vi "ExecuteCommand.vi"(8 "error in (no error)":errorcluster, 10 "Command":string, 11 "VISA resource name":refnum<visa-resource-name>) -> (0 "error out":errorcluster, 2 "Response":string, 3 "VISA resource name out":refnum<visa-resource-name>)   [LabVIEW 2018, in "CAEN PSM.lvlib"]
uses:
  CAEN PSM.lvlib
  <vilib>/Instr/_visa.llb/Select Event Type.ctl
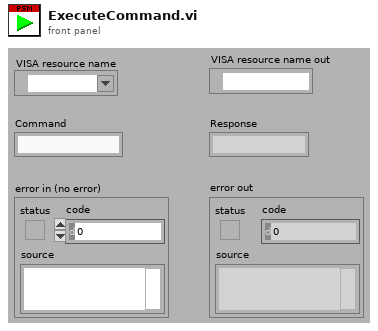
[diagram p1: front panel]
types:
  T1 = typedef "Select Event Type.ctl" = u32
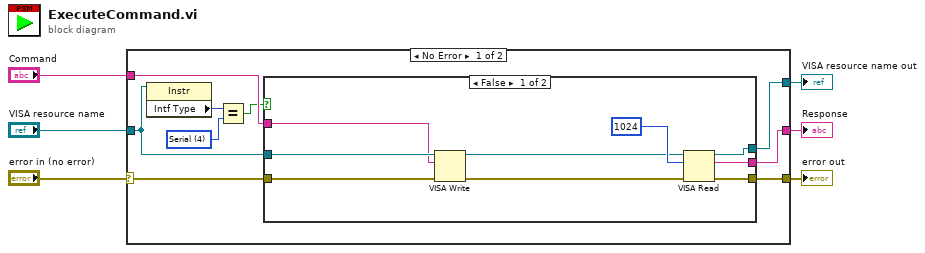
[diagram p0: block diagram]
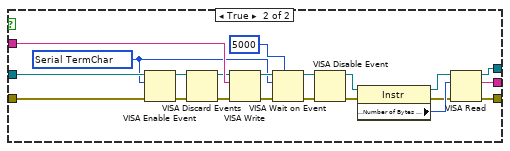
[diagram p2: hidden frame]
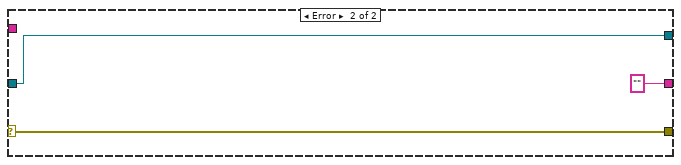
[diagram p3: hidden frame]
diagram:
  n1 = case shown="No Error" "error in (no error)" {
    selector: "error in (no error)" -> [w12 w48]
    tunnel: "Command" -> [w11 _]
    tunnel: "VISA resource name" -> [w10 w46]
    tunnel: [w15 "" ("read buffer")] -> w4
    tunnel: [w14 w48] -> w3
    tunnel: [w13 w46] -> w2
    frame No Error {
      w8 = u16 4 items=["GPIB"=1, "VXI"=2, "GPIB-VXI"=3, "Serial"=4, "PXI"=5, "TCPIP"=6, "USB"=7] ("Interface Information:Interface Type")
      n2 = property class="Instr"(reference=w10) -> ("Intf Type"=w9:u16)  [unwired: 1 in, 2 out]
      n3 = Equal?(x=w9, y=w8) -> (x = y?=w7:bool)
      n4 = case shown="False" w7 {
        tunnel: [w20 w43] -> w15
        tunnel: [w21 w42] -> w14
        tunnel: [w19 w41] -> w13
        tunnel: w10 -> [w23 w34]
        tunnel: w12 -> [w24 w33]
        tunnel: w11 -> [w17 w32]
        frame False {
          n5 = VISA Write(VISA resource name=w23, write buffer=w17, error in (no error)=w24) -> (VISA resource name out=w16:refnum<visa-resource-name>, error out=w22:errorcluster)  [unwired: 1 out]
          n6 = VISA Read(VISA resource name=w16, byte count=u32 1024, error in (no error)=w22) -> (VISA resource name out=w19:refnum<visa-resource-name>, read buffer=w20:string, error out=w21:errorcluster)  [unwired: 1 out]
        }
        frame True {
          w25 = T1 1073684516 items=["Service Request"=1073684491, "Trigger"=3221168138, "Clear"=1073684493, "VXI Signal"=1073684512, "VXI/VME Interrupt"=3221168161, "VXI/VME Sysfail"=1073684509, "VXI/VME Sysreset"=1073684510, "GPIB CIC"=1073684498, "GPIB Talk"=1073684499, "GPIB Listen"=1073684500, "PXI Interrupt"=1073684514, "Serial Break"=1073684515, "Serial TermChar"=1073684516, "Serial CTS"=1073684521, "Serial DSR"=1073684522, "Serial DCD"=1073684524, "Serial RI"=1073684526, "Serial Character"=1073684533, "USB Interrupt"=1073684535, "All Enabled"=1073709055] ("Event Type")
          n7 = VISA Enable Event(8:w33, 10:w25, 11:w34) -> (0:w30:errorcluster, 3:w31:refnum<visa-resource-name>)  [unwired: 1 in]
          n8 = VISA Discard Events(8:w30, 11:w31) -> (0:w28:errorcluster, 3:w29:refnum<visa-resource-name>)  [unwired: 2 in]
          n9 = VISA Write(VISA resource name=w29, write buffer=w32, error in (no error)=w28) -> (VISA resource name out=w27:refnum<visa-resource-name>, error out=w26:errorcluster)  [unwired: 1 out]
          n10 = VISA Wait on Event(7:u32 5000 ("timeout (0)"), 8:w26, 10:w25, 11:w27) -> (0:w39:errorcluster, 3:w38:refnum<visa-resource-name>)  [unwired: 1 in, 2 out]
          n11 = VISA Disable Event(8:w39, 11:w38) -> (0:w45:errorcluster, 3:w44:refnum<visa-resource-name>)  [unwired: 2 in]
          n12 = property class="Instr"(reference=w44, error in=w45) -> (reference out=w36:refnum<visa-resource-name>, error out=w35:errorcluster, "Serial Settings:Number of Bytes at Serial Port"=w37:u32)
          n13 = VISA Read(VISA resource name=w36, byte count=w37, error in (no error)=w35) -> (VISA resource name out=w41:refnum<visa-resource-name>, read buffer=w43:string, error out=w42:errorcluster)  [unwired: 1 out]
        }
      }
    }
    frame Error {
    }
  }
  "Response" <- w4
  "error out" <- w3
  "VISA resource name out" <- w2
